vi "Teleop.vi"(10 "Match Info":T1={"Autonomous Elapsed Seconds"=0.0, "TeleOp Elapsed Seconds"=0.0, "Disabled Elapsed Seconds"=0.0, "Visited Autonomous"=FALSE, "Visited TeleOp"=FALSE, "Visited Disabled"=FALSE, "Autonomous Settings"={"Autonomous Style"=enum."Independent", "VI Refnum"=refnum}}, 11 "Call Context":T2) -> ()   [LabVIEW 2015]
doc: "This VI is called for each TeleOp packet received from the DS where the robot is not disabled. It is often used to read from the joysticks and update I/O or to update setpoints for timed control loops. It should complete and return within 20 milliseconds or it may miss DS packets."
uses:
  <vilib>/Rock Robotics/WPI/DriverStation/WPI_DriverStationDerivedRobotMode.ctl
  <vilib>/Rock Robotics/WPI/DriverStation/WPI_DriverStationMatch Info.ctl
  RefnameEnum.ctl
  LEDSaction.ctl
  Robot Global Data.vi
  <vilib>/Rock Robotics/WPI/Joystick/WPI_JoystickGetSetRefNum.vi
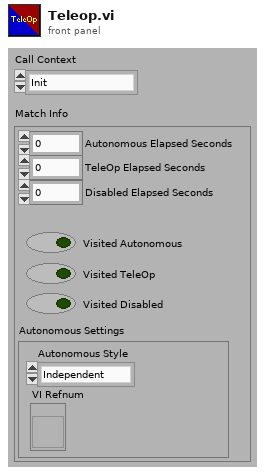
[diagram p1: front panel]
types:
  T1 = typedef "WPI_DriverStationMatch Info.ctl" = cluster{"Autonomous Elapsed Seconds":dbl, "TeleOp Elapsed Seconds":dbl, "Disabled Elapsed Seconds":dbl, "Visited Autonomous":bool, "Visited TeleOp":bool, "Visited Disabled":bool, "Autonomous Settings":cluster{"Autonomous Style":enum16{"Iterative", "Independent"}, "VI Refnum":refnum<vi>}}
  T2 = typedef "WPI_DriverStationDerivedRobotMode.ctl" = enum16{"Init", "Execute", "Stop"}
  T3 = typedef "RefnameEnum.ctl" = enum16{"TankDrive", "Controller1", "Controller2", "SonicShifter", "Compressor"}
  T4 = typedef "WPI_JoystickDevRef.ctl" = cluster{"Device":T5}
  T5 = typedef "WPI_JoystickDeviceEnum.ctl" = enum16{"USB 0", "USB 1", "USB 2", "USB 3", "USB 4", "USB 5"}
  T6 = cluster{"Button 1":bool, "Button 2":bool, "Button 3":bool, "Button 4":bool, "Button 5":bool, "Button 6":bool, "Button 7":bool, "Button 8":bool, "Button 9":bool, "Button 10":bool, "Button 11":bool, "Button 12":bool}
  T7 = cluster{"axis 1 (x)":dbl, "axis 2 (y)":dbl, "axis 3 (throttle)":dbl, "axis 4":dbl, "axis 5":dbl, "axis 6":dbl}
  T8 = typedef "LEDSaction.ctl" = enum16{"Init", "10SecondsLeft", "LimitDown", "LimitUp", "CollectDown", "CollectUp", "NotHot", "Hot", "Shift", "RollBack", "RollFwd", "Shoot", "Distance Low", "DistanceHigh", "PressureLow", "PressureHigh"}
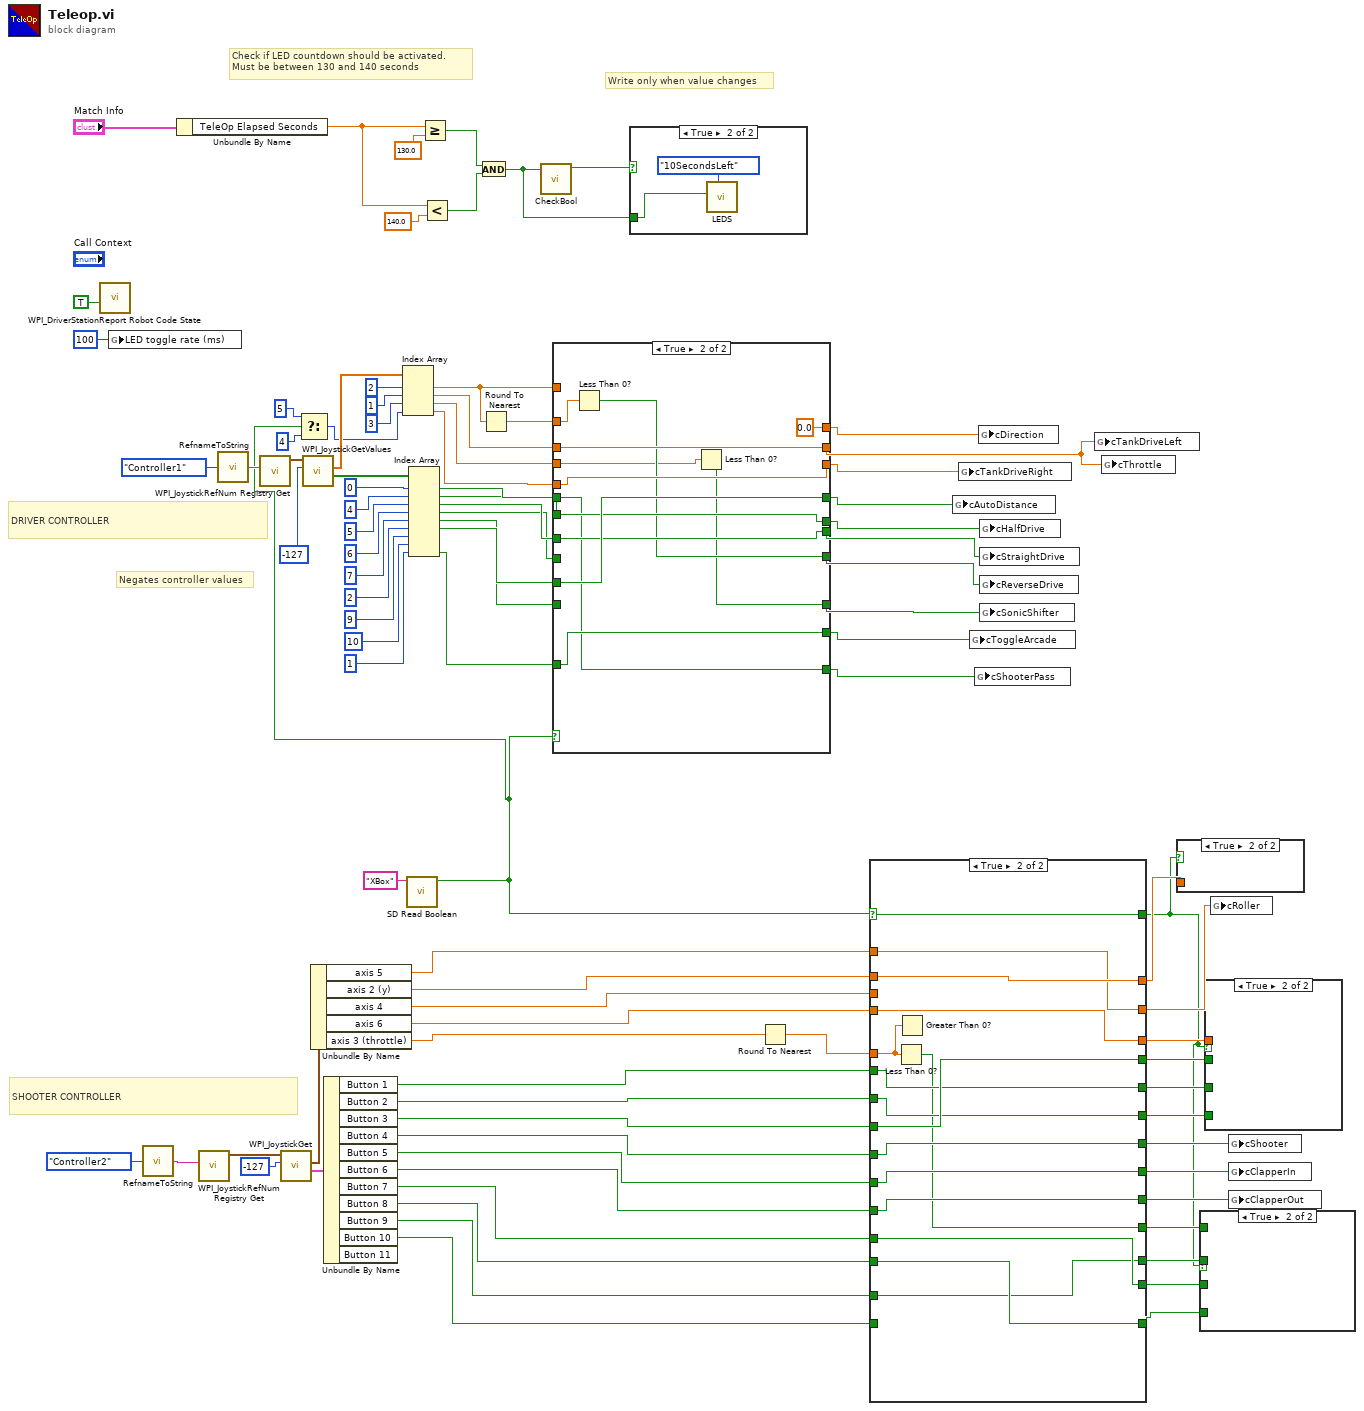
[diagram p0: block diagram]
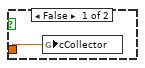
[diagram p2: hidden frame]
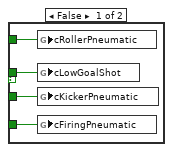
[diagram p3: hidden frame]
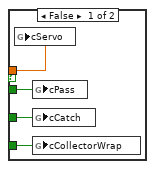
[diagram p4: hidden frame]
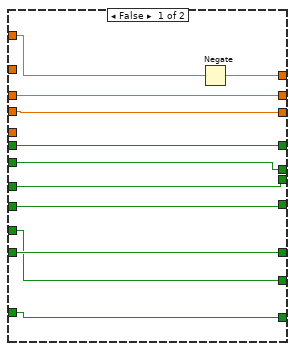
[diagram p6: hidden frame]
diagram:
  # "Write only when value changes"
  # "Check if LED countdown should be activated.\nMust be between 130 and 140 seconds"
  # "SHOOTER CONTROLLER"
  # "DRIVER CONTROLLER"
  # "Negates controller values"
  n1 = call <vilib>:"WPI_DriverStationReport Robot Code State.vi"("TeleOp"=TRUE ("Autonomous")) -> ()  [unwired: 10 in, 1 out]
  n2 = global write "Robot Global Data.vi" "LED toggle rate (ms)"(u32 100 ("LED ms toggle rate")) -> ()
  n3 = call "RefnameToString.vi"("Enum"=RefnameEnum."Controller2") -> ("Refname"=w86:string)
  n4 = Unbundle By Name("Match Info") -> ("TeleOp Elapsed Seconds"=w39:dbl)
  n5 = call <vilib>:"WPI_JoystickRefNum Registry Get.vi"("refnum name"=w86) -> ("JoystickDevRef"=w84:T4)  [unwired: 1 in, 9 out]
  n6 = call "RefnameToString.vi"("Enum"=RefnameEnum."Controller1") -> ("Refname"=w89:string)
  n7 = call <vilib>:"WPI_JoystickRefNum Registry Get.vi"("refnum name"=w89) -> ("JoystickDevRef"=w32:T4)  [unwired: 1 in, 9 out]
  n8 = call <vilib>:"WPI_JoystickGet.vi"("Scaler"=i8 -127, "JoystickDevRef"=w84) -> ("Buttons"=w82:T6, "Axes"=w83:T7)  [unwired: 4 out]
  n9 = call <vilib>:"WPI_JoystickGetValues.vi"("Scaler"=i8 -127, "JoystickDevRef"=w32) -> ("Buttons"=w25:bool[], "Axes"=w30:dbl[])  [unwired: 5 in, 3 out]
  n10 = Unbundle By Name(w83) -> ("axis 5"=w54:dbl, "axis 2 (y)"=w62:dbl, "axis 4"=w61:dbl, "axis 6"=w60:dbl, "axis 3 (throttle)"=w59:dbl)
  n11 = Unbundle By Name(w82) -> ("Button 1"=w78:bool, "Button 2"=w79:bool, "Button 3"=w80:bool, "Button 4"=w81:bool, "Button 5"=w77:bool, "Button 6"=w76:bool, "Button 7"=w75:bool, "Button 8"=w63:bool, "Button 9"=w74:bool, "Button 10"=w73:bool)  [unwired: 1 out]
  n12 = call <vilib>:"SD Read Boolean.vi"("Name"="XBox") -> ("Boolean"=w5:bool)  [unwired: 8 in, 2 out]
  n13 = Select(t=5 ("index"), s=w5, f=4 ("index")) -> (s? t:f=w4:i32)
  n14 = Index Array(array=w30, index #1=2 ("index"), index #2=1 ("index"), index #3=3 ("index"), index #4=w4) -> (element #1=w29:dbl, element #2=w28:dbl, element #3=w27:dbl, element #4=w26:dbl)
  n15 = Index Array(array=w25, index #1=0 ("index"), index #2=4 ("index"), index #3=5 ("index"), index #4=6 ("index"), index #5=7 ("index"), index #6=2 ("index"), index #7=9 ("index"), index #8=10 ("index"), index #9=1 ("index")) -> (element #1=w15:bool, element #2=w14:bool, element #3=w13:bool, element #4=w12:bool, element #5=w10:bool, element #6=w11:bool, element #9=w9:bool)  [unwired: 2 out]
  n16 = Greater Or Equal?(x=w39, y=130.0) -> (x >= y?=w37:bool)
  n17 = Less?(x=w39, y=140.0) -> (x < y?=w36:bool)
  n18 = And(x=w37, y=w36) -> (x .and. y?=w34:bool)
  n19 = Round To Nearest(number=w29) -> (nearest integer value=w48:dbl)
  n20 = call "CheckBool.vi"("Input Boolean"=w34) -> ("Boolean Changed?"=w35:bool)  [unwired: 10 in]
  n21 = case shown="True" w5 {
    tunnel: w28 -> [w102 w113]
    tunnel: [w102 w113] -> w44
    tunnel: w27 -> [w101 w105]
    tunnel: [w101 w114] -> w43
    tunnel: [w100 w112] -> w53
    tunnel: w15 -> [w100 w106]
    tunnel: [w99 w111] -> w52
    tunnel: w14 -> [w99 w111]
    tunnel: [w98 w110] -> w51
    tunnel: w13 -> [w98 w110]
    tunnel: w12 -> [w97 _]
    tunnel: [w97 w109] -> w50
    tunnel: [w96 w104] -> w49
    tunnel: w10 -> [w96 _]
    tunnel: w26 -> [_ w114]
    tunnel: w11 -> [w94 w112]
    tunnel: w48 -> [_ w108]
    tunnel: [w93 0.0] -> w45
    tunnel: w29 -> [w95 _]
    tunnel: [w94 w107] -> w47
    tunnel: w9 -> [w92 w107]
    tunnel: [w92 w106] -> w33
    frame False {
      n22 = Negate(x=w95) -> (-x=w93:dbl)
    }
    frame True {
      n23 = Less Than 0?(x=w108) -> (x < 0?=w109:bool)
      n24 = Less Than 0?(x=w105) -> (x < 0?=w104:bool)
    }
  }
  n25 = case shown="True" w35 {
    tunnel: w34 -> [_ w115]
    frame False {
    }
    frame True {
      n26 = call "LEDS.vi"("Action"=LEDSaction."10SecondsLeft", "On/Off"=w115) -> ()  [unwired: 9 in, 1 out]
    }
  }
  n27 = Round To Nearest(number=w59) -> (nearest integer value=w58:dbl)
  n28 = case shown="True" w5 {
    selector: w5 -> [w117 w131]
    tunnel: w81 -> [w125 w142]
    tunnel: w80 -> [w124 w145]
    tunnel: w79 -> [w123 w143]
    tunnel: w78 -> [w122 w144]
    tunnel: w77 -> [w126 w141]
    tunnel: w76 -> [w127 w140]
    tunnel: w75 -> [w128 w139]
    tunnel: w74 -> [w129 w132]
    tunnel: w73 -> [w130 _]
    tunnel: [w130 w138] -> w72
    tunnel: [w129 w139] -> w71
    tunnel: [w128 w134] -> w70
    tunnel: [w127 w140] -> w69
    tunnel: [w126 w141] -> w68
    tunnel: [w125 w142] -> w67
    tunnel: [w124 w143] -> w66
    tunnel: [w123 w144] -> w65
    tunnel: [w122 w145] -> w64
    tunnel: w63 -> [w118 w138]
    tunnel: [w121 w137] -> w57
    tunnel: w62 -> [w121 w137]
    tunnel: w61 -> [w120 _]
    tunnel: [w120 w135] -> w56
    tunnel: w60 -> [w119 w136]
    tunnel: [w119 w136] -> w55
    tunnel: w58 -> [_ w133]
    tunnel: w54 -> [_ w135]
    tunnel: [w118 w132] -> w42
    tunnel: [w117 w131] -> w1
    frame False {
    }
    frame True {
      n29 = Less Than 0?(x=w133) -> (x < 0?=w134:bool)
      n30 = Greater Than 0?(x=w133) -> ()  [unwired: 1 out]
    }
  }
  n31 = global write "Robot Global Data.vi" "cAutoDistance"(w53) -> ()
  n32 = global write "Robot Global Data.vi" "cTankDriveRight"(w43) -> ()
  n33 = global write "Robot Global Data.vi" "cToggleArcade"(w47) -> ()
  n34 = global write "Robot Global Data.vi" "cShooterPass"(w33) -> ()
  n35 = global write "Robot Global Data.vi" "cDirection"(w45) -> ()
  n36 = global write "Robot Global Data.vi" "cHalfDrive"(w52) -> ()
  n37 = global write "Robot Global Data.vi" "cStraightDrive"(w51) -> ()
  n38 = global write "Robot Global Data.vi" "cReverseDrive"(w50) -> ()
  n39 = global write "Robot Global Data.vi" "cSonicShifter"(w49) -> ()
  n40 = global write "Robot Global Data.vi" "cTankDriveLeft"(w44) -> ()
  n41 = global write "Robot Global Data.vi" "cThrottle"(w44) -> ()
  n42 = case shown="True" w1 {
    tunnel: w57 -> [w146 _]
    frame False {
      n43 = global write "Robot Global Data.vi" "cCollector"(w146) -> ()
    }
    frame True {
    }
  }
  n44 = case shown="True" w1 {
    tunnel: w72 -> [w150 _]
    tunnel: w71 -> [w149 _]
    tunnel: w70 -> [w148 _]
    tunnel: w42 -> [w147 _]
    frame False {
      n45 = global write "Robot Global Data.vi" "cRollerPneumatic"(w148) -> ()
      n46 = global write "Robot Global Data.vi" "cLowGoalShot"(w147) -> ()
      n47 = global write "Robot Global Data.vi" "cKickerPneumatic"(w149) -> ()
      n48 = global write "Robot Global Data.vi" "cFiringPneumatic"(w150) -> ()
    }
    frame True {
    }
  }
  n49 = case shown="True" w1 {
    tunnel: w66 -> [w154 _]
    tunnel: w65 -> [w153 _]
    tunnel: w64 -> [w152 _]
    tunnel: w55 -> [w151 _]
    frame False {
      n50 = global write "Robot Global Data.vi" "cServo"(w151) -> ()
      n51 = global write "Robot Global Data.vi" "cPass"(w152) -> ()
      n52 = global write "Robot Global Data.vi" "cCatch"(w153) -> ()
      n53 = global write "Robot Global Data.vi" "cCollectorWrap"(w154) -> ()
    }
    frame True {
    }
  }
  n54 = global write "Robot Global Data.vi" "cRoller"(w56) -> ()
  n55 = global write "Robot Global Data.vi" "cShooter"(w67) -> ()
  n56 = global write "Robot Global Data.vi" "cClapperIn"(w68) -> ()
  n57 = global write "Robot Global Data.vi" "cClapperOut"(w69) -> ()
